vi "Scan I2C Bus.vi"(8 "error in (no error)":errorcluster, 10 "Serial Input":string, 11 "FPGA Ref":refnum<k20>) -> (0 "error out":errorcluster, 3 "Scanned Addresses":i32[](array[numeric]))   [LabVIEW 2025, in "I2C Bus Monitor.lvclass"]
uses:
  I2C Bus Monitor.lvclass
  I2C Bus Monitor.lvclass/I2C Bus Monitor.ctl
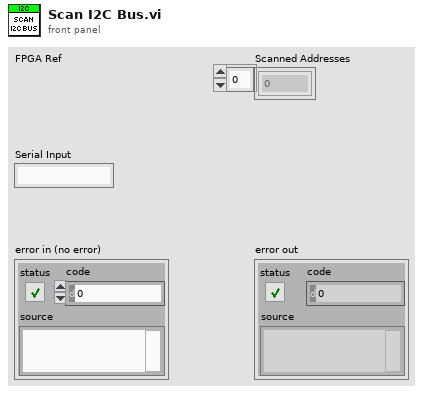
[diagram p1: front panel]
types:
  T1 = cluster{"Serial Channel":string, "Slave Address":u8, "Register Address":u16, "Data":u8, "Write":bool}
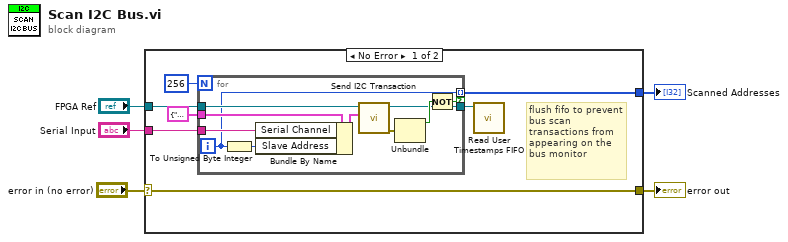
[diagram p0: block diagram]
diagram:
  n1 = case shown="No Error" "error in (no error)" {
    selector: "error in (no error)" -> [w6 w23]
    tunnel: [w11 _] -> w5
    tunnel: "FPGA Ref" -> [w8 _]
    tunnel: "Serial Input" -> [w7 _]
    tunnel: [w6 w23] -> w1
    frame No Error {
      # "flush fifo to prevent bus scan transactions from appearing on the bus monitor"
      n2 = for {
        N: 256 -> [_]
        tunnel: w8 -> [w22]
        tunnel: [w16] -> w11 mode=indexing if=w18
        tunnel: T1 {"Serial Channel"="", "Slave Address"=0, "Register Address"=0, "Data"=0, "Write"=FALSE} ("I2C Command") -> [w21]
        tunnel: w7 -> [w19]
        tunnel: [w14] -> w12
        i -> [w16]
        n3 = To Unsigned Byte Integer(number=w16) -> (unsigned 8bit integer=w15:u8)
        n4 = Bundle By Name(cluster=w21, "Serial Channel"=w19, "Slave Address"=w15) -> (w20:T1)
        n5 = call "Send I2C Transaction.vi"("I2C Command"=w20, "FPGA Ref in"=w22) -> ("Error Out"=w13:errorcluster, "FPGA Ref out"=w14:refnum<k20>)  [unwired: 7 in, 1 out]
        n6 = Unbundle(w13) -> ("status"=w17:bool)  [unwired: 2 out]
        n7 = Not(x=w17) -> (.not. x?=w18:bool)
      }
      n8 = call "Read User Timestamps FIFO.vi"("FPGA Ref in"=w12) -> ()  [unwired: 7 in, 4 out]
    }
    frame Error {
    }
  }
  "Scanned Addresses" <- w5
  "error out" <- w1
